vi "kAverager.vi"(8 "Avg Len":i32, 11 "Input":dbl) -> (3 "Avg":dbl)   [LabVIEW 2010, in "KevLib01.lvlib"]
uses:
  KevLib01.lvlib
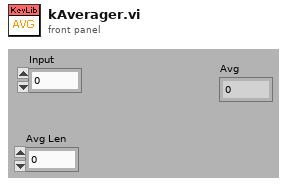
[diagram p1: front panel]
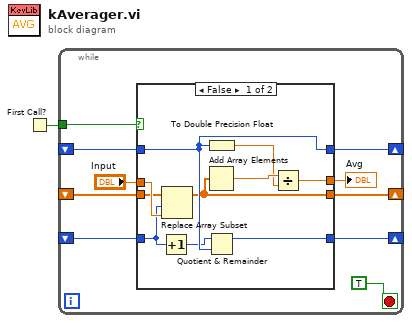
[diagram p0: block diagram]
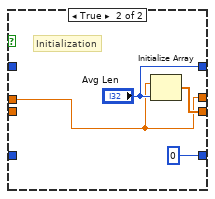
[diagram p2: hidden frame]
diagram:
  n1 = First Call?() -> (First Call?: T/F=w1:bool)
  n2 = while {
    tunnel: w1 -> [w10]
    shift-right: [w9] -> _
    shift-left: _ -> [w6]
    shift-right: [w8] -> _
    shift-left: _ -> [w5]
    shift-right: [w7] -> _
    shift-left: _ -> [w4]
    stop <- TRUE stop-if-true
    n3 = case shown="False" w10 {
      tunnel: [w15 w23] -> w9
      tunnel: [w19 "Avg Len"] -> w8
      tunnel: [w13 0 ("index")] -> w7
      tunnel: w6 -> [w16 _]
      tunnel: w5 -> [w19 _]
      tunnel: w4 -> [w12 _]
      tunnel: "Input" -> [w18 w22]
      tunnel: [w14 w22] -> w2
      frame False {
        n4 = Increment(x=w12) -> (x+1=w17:i32)
        n5 = Replace Array Subset(array=w16, new element=w18, index=w12) -> (w15:dbl[])
        n6 = Add Array Elements(numeric array=w15) -> (sum=w21:dbl)
        n7 = To Double Precision Float(number=w19) -> (double precision float=w20:dbl)
        n8 = Quotient & Remainder(x=w17, y=w19) -> (x-y*floor(x/y)=w13:i32)  [unwired: 1 out]
        n9 = Divide(x=w21, y=w20) -> (x/y=w14:dbl)
      }
      frame True {
        # "Initialization"
        n10 = Initialize Array(w22, "Avg Len") -> (w23:dbl[])
      }
    }
    "Avg" <- w2
  }
